vi "Configure Sample RateI.vi"(8 "error in":errorcluster, 9 "Samples per Second":i32=10 min=1 max=10000000, 11 "VISA resource name":refnum<visa-resource-name>) -> (0 "error out":errorcluster, 3 "VISA resource name out":refnum<visa-resource-name>)   [LabVIEW 2020, in "BDAQ-6104.lvlib"]
doc: "Configure the sample rate for streaming analog channel data."
uses:
  <instrlib>/BDAQ-6104/BDAQ-6104.lvlib
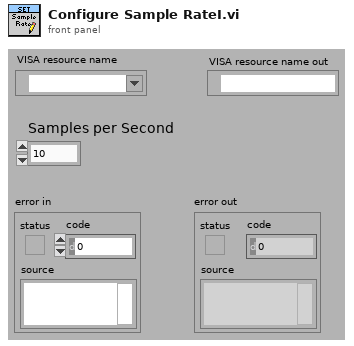
[diagram p1: front panel]
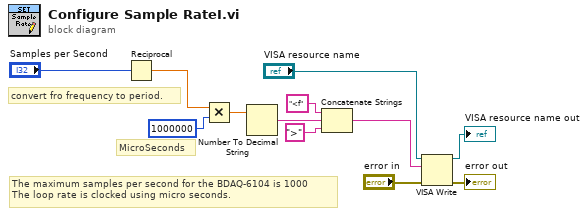
[diagram p0: block diagram]
diagram:
  # "convert fro frequency to period."
  # "MicroSeconds"
  # "The maximum samples per second for the BDAQ-6104 is 1000\nThe loop rate is clocked using micro seconds."
  n1 = Reciprocal(x="Samples per Second") -> (1/x=w1:dbl)
  n2 = Multiply(x=w1, y=1000000) -> (x*y=w3:dbl)
  n3 = Number To Decimal String(number=w3) -> (decimal integer string=w10:string)  [unwired: 1 in]
  n4 = Concatenate Strings("<f", w10, ">") -> (w9:string)
  n5 = VISA Write(VISA resource name="VISA resource name", write buffer=w9, error in (no error)="error in") -> (VISA resource name out=→"VISA resource name out":refnum<visa-resource-name>, error out=→"error out":errorcluster)  [unwired: 1 out]
